vi "MALT Get Several.vi"(8 "error in":errorcluster, 9 "Block":i32, 10 "Address":i32, 11 "MALT CardType":T1=enum."MALT132") -> (0 "error out":errorcluster, 3 "Status":u8[](array[numeric]) format="%02x")   [LabVIEW 2018]
uses:
  Types/MALT CardTypes.ctl
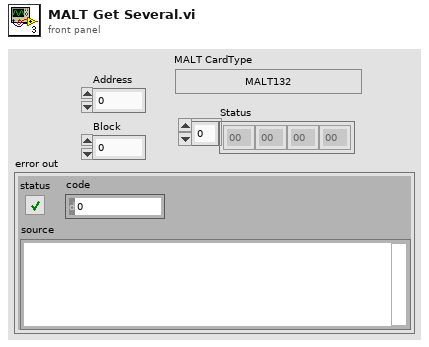
[diagram p1: front panel]
types:
  T1 = typedef "MALT CardTypes.ctl" = enum32{"-", "YAV90832", "YAV904X8", "MALT132", "YAV91616", "YAV90PIN", "YAV90096", "YAV90HVT", "YAV90CLR", "YAV90128", "YAV90PNE", "YAVCANCON", "YAV91775", "YAV90XXX", "YAV90MMU", "H730050", "H710060", "H710061", "YAV90304", "MMI", "YAV90060", "YAV90MUX", "YAV90059", "Not Defined"}
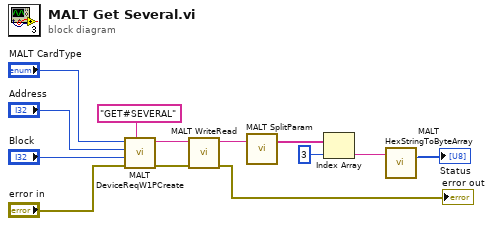
[diagram p0: block diagram]
diagram:
  n1 = call "MALT DeviceReqW1PCreate.vi"("Cmd"="GET#SEVERAL" ("cmd"), "error in"="error in", "Param1"="Block", "Address"="Address", "CardType"="MALT CardType") -> ("error out"=w5:errorcluster, "Request"=w9:string)  [unwired: 5 in]
  n2 = call "MALT WriteRead.vi"("error in"=w5, "Request"=w9) -> ("error out"=→"error out":errorcluster, "Response"=w13:string)  [unwired: 8 in]
  n3 = call "MALT SplitParam.vi"("Line"=w13) -> ("Items"=w11:string[])  [unwired: 2 in]
  n4 = Index Array(array=w11, index=3) -> (element=w2:string)
  n5 = call "MALT HexStringToByteArray.vi"("String in"=w2) -> ("Bytes out"=→"Status":u8[])  [unwired: 2 in]
